vi "UI Main.vi"() -> ()   [LabVIEW 2018]
doc: "This is the main user interface for the LabVIEW Real-Time Sequencer."
uses:
  controls/UI Data.ctl
  controls/Configured Step.ctl
  controls/VI Reference Type.ctl
  controls/FPGA State.ctl
  Globals/Global - All UI Loop Stop.vi
  Globals/Global - UI Stream and Variable Connections.vi
  Globals/Global - Configuration Options.vi
  support/User Event - Stop/User Event - Stop.lvlib
  support/Message Queue/Message Queue.lvlib
panel:
  in  "Switch to Safe State":bool
  in  "Exit":bool
  out "System Status":string
  out "Current FPGA Control Mode":u16(ring) items=["Safe State", "Control (PID)"]
  in  "Settings Tab":T1(tab)
  in  "Build Sequence":bool
  in  "Control Sequence":i32(listbox)
  in  "Stop Sequence":bool
  in  "Pause":bool
  in  "Start":bool
  out "Output Values":cluster{dbl, dbl}(graph)
  out "Input Values":cluster{dbl, dbl}(graph)
  out "Actual Loop Period (ticks)":u32
  out "Largest Contiguous Memory (bytes)":dbl(graph)
  out "CPU Usage (%)":dbl(graph)
  out "Connected?":bool
  in  "Connect to Controller":bool
  in  "Controller Address":string
  # "LabVIEW Real-Time Sequencer"
  # "Connection Settings"
  # "Step Configuration Preview"
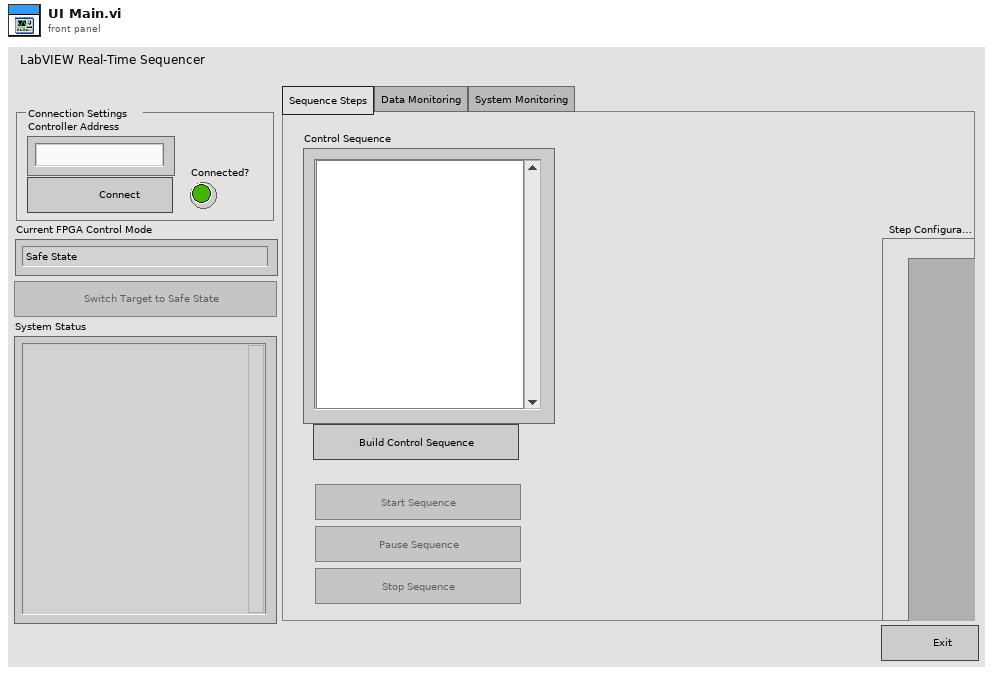
[diagram p1: front panel]
types:
  T1 = enum32{"Sequence Steps", "Data Monitoring", "System Monitoring"}
  T2 = typedef "VI Reference Type.ctl" = refnum<vi>
  T3 = typedef "Configured Step.ctl" = cluster{"Step Name":string, "Value":variant}
  T4 = typedef "UI Data.ctl" = cluster{"Switch to Safe State Ref":refnum<vi>, "Start Sequence Ref":refnum<vi>, "Pause Sequence Ref":refnum<vi>, "Stop Sequence Ref":refnum<vi>, "Build Sequence Ref":refnum<vi>, "SubPanel Ref":refnum<vi>}
  T5 = typedef "Message Queue.lvlib/All Message Queues.ctl" = cluster{"Sequencer Cmd Queue":refnum<queue>, "Vision Cmd Queue":refnum<queue>, "Motion Cmd Queue":refnum<queue>, "Message Handling Queue":refnum<queue>}
  T6 = typedef "FPGA State.ctl" = enum16{"Safe State", "Control (PID)"}
  T7 = typedef "Variable References.ctl" = cluster{"CPU Usage":refnum<k21>, "Contiguous Memory":refnum<k21>, "Input Values":refnum<k21>, "Output Values":refnum<k21>, "FPGA Mode":refnum<k21>, "Actual Loop Period":refnum<k21>}
  T8 = typedef "Raw Values.ctl" = cluster{"Channel 0":fxp<+/-,20,5>, "Channel 1":fxp<+/-,20,5>, "Channel 2":bool}
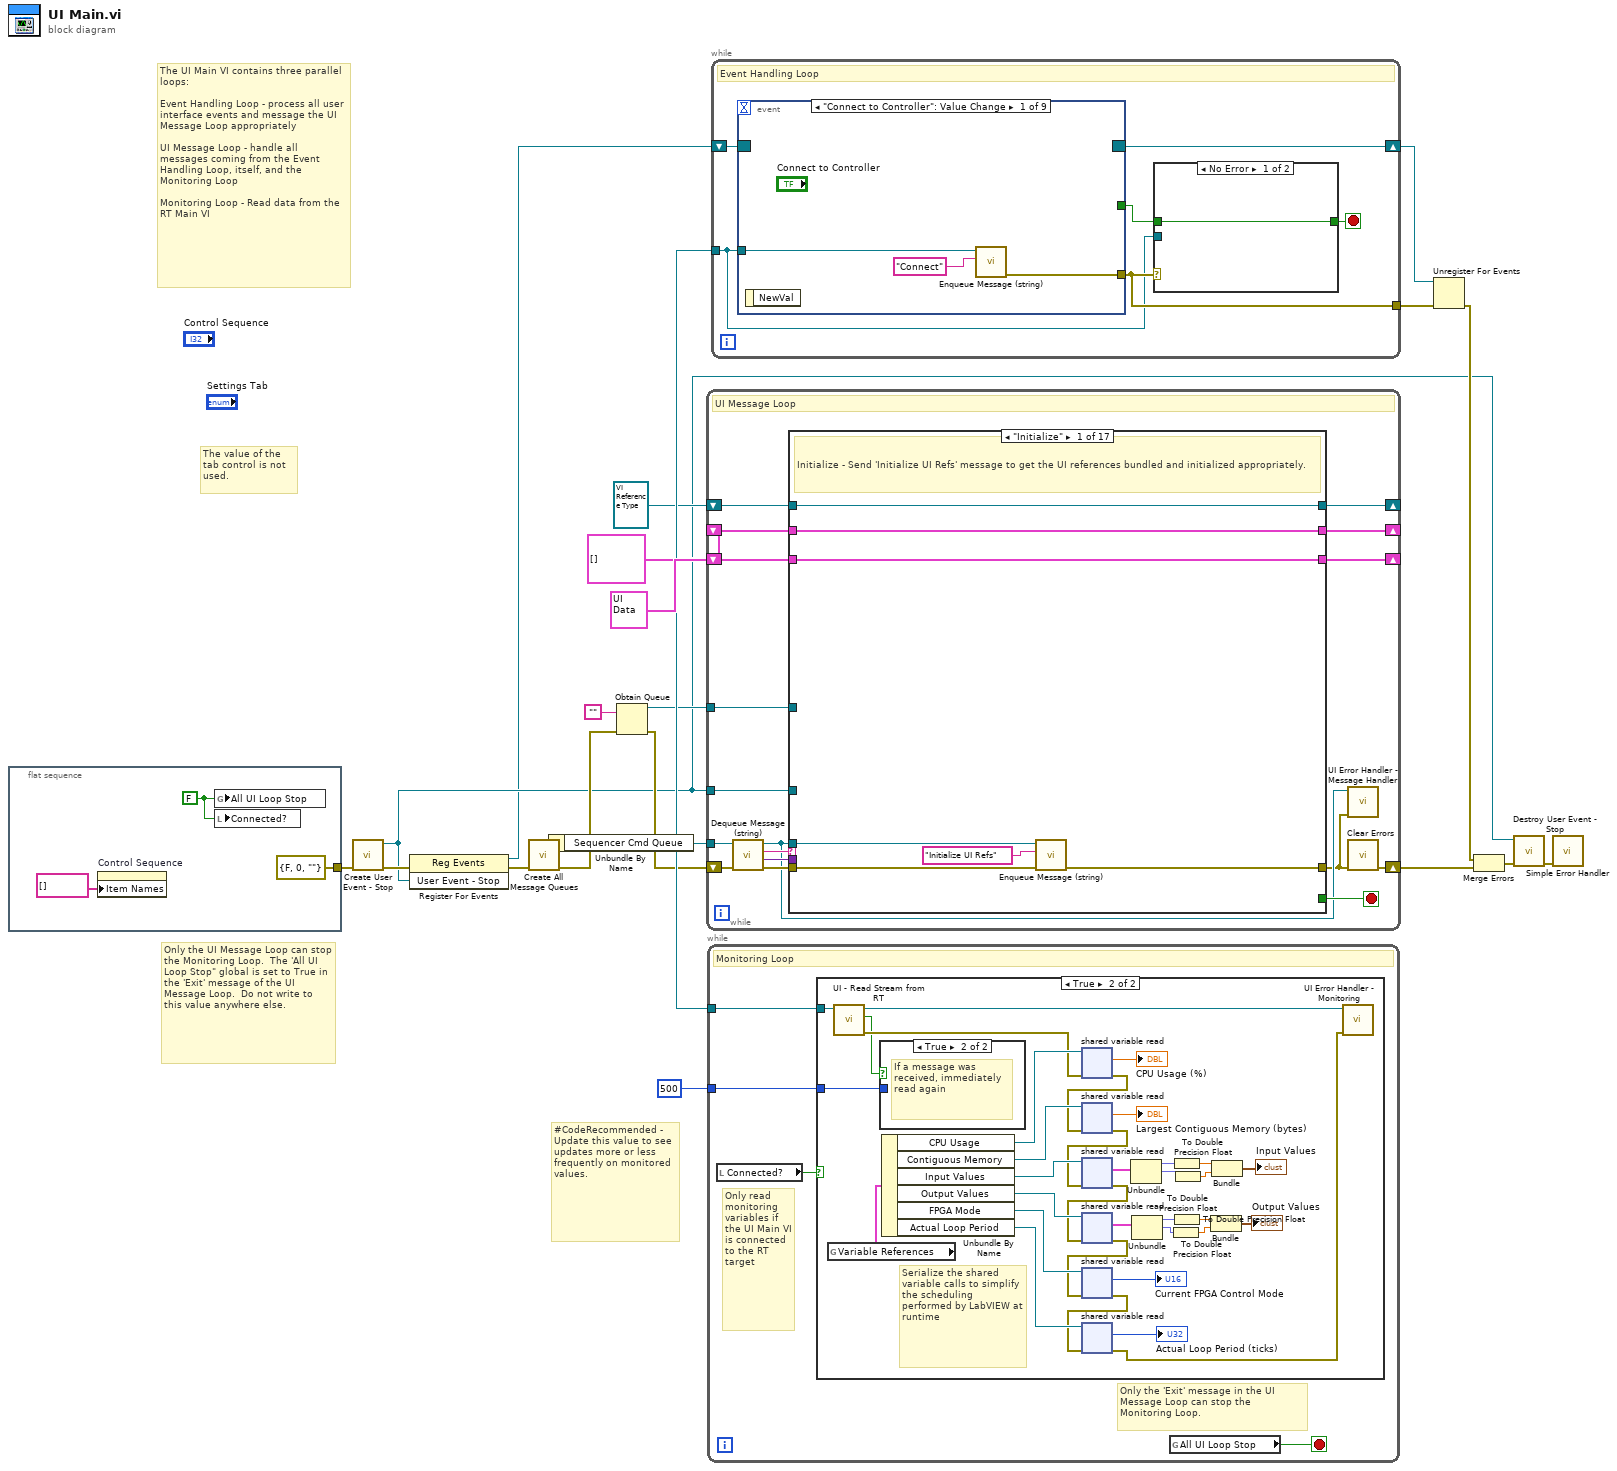
[diagram p0: block diagram]
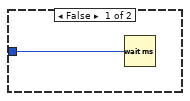
[diagram p2: hidden frame]
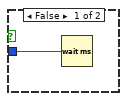
[diagram p3: hidden frame]
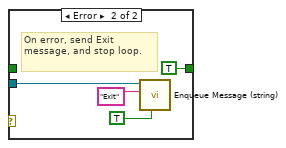
[diagram p4: hidden frame]
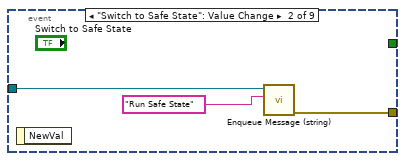
[diagram p5: hidden frame]
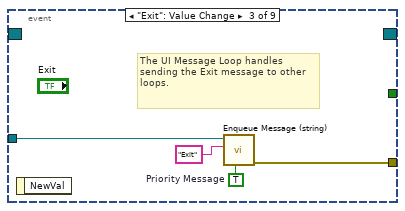
[diagram p6: hidden frame]
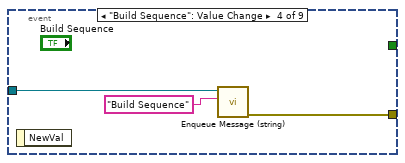
[diagram p7: hidden frame]
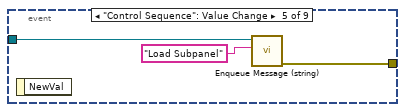
[diagram p8: hidden frame]
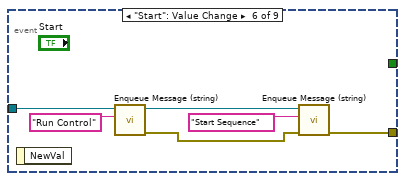
[diagram p9: hidden frame]
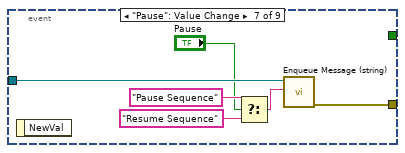
[diagram p10: hidden frame]
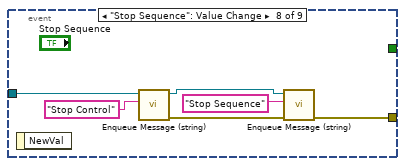
[diagram p11: hidden frame]
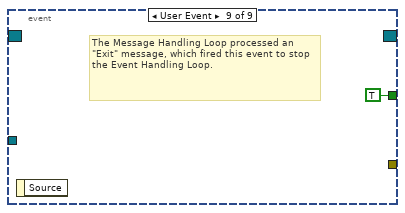
[diagram p12: hidden frame]
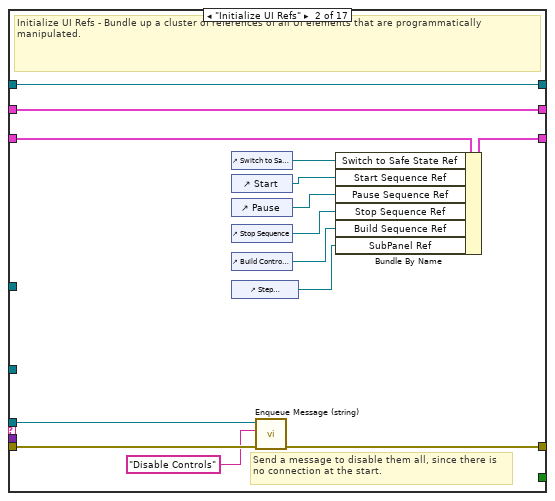
[diagram p13: hidden frame]
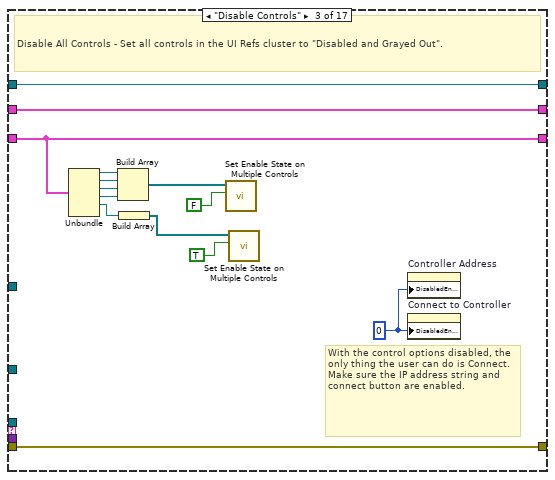
[diagram p14: hidden frame]
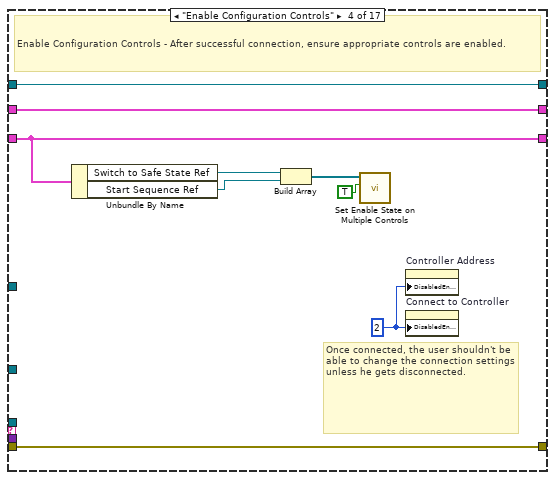
[diagram p15: hidden frame]
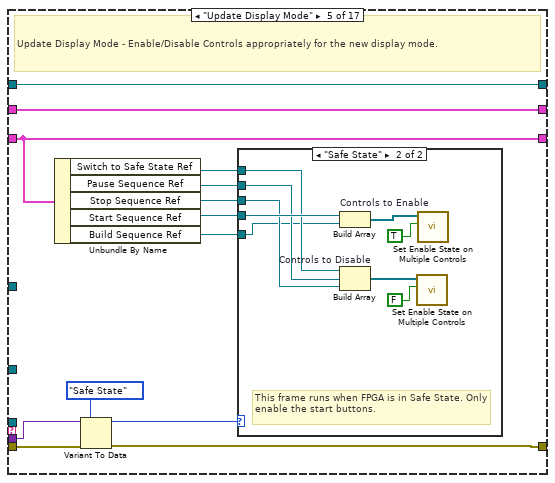
[diagram p16: hidden frame]
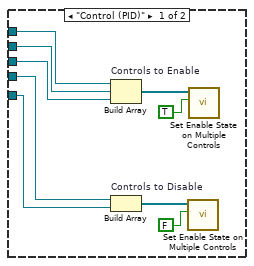
[diagram p17: hidden frame]
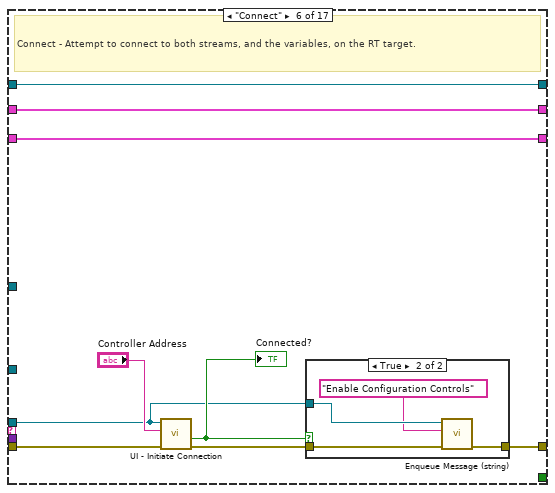
[diagram p18: hidden frame]
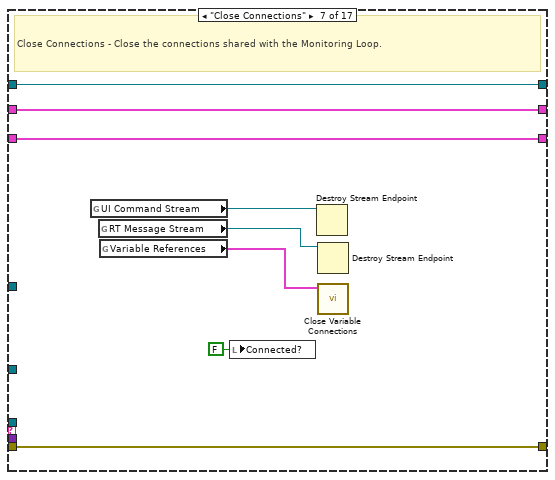
[diagram p20: hidden frame]
diagram:
  # "#CodeRecommended - Update this value to see updates more or less frequently on monitored values."
  # "The UI Main VI contains three parallel loops:\n\nEvent Handling Loop - process all user interface events and message the UI Message Loop appropriately\n\nUI Message Loop - handle all messages coming from the Event Handling Loop, itself, and the Monitoring Loop\n\nMonitoring Loop - Read data from the RT Main VI"
  # "The value of the tab control is not used."
  # "Only the UI Message Loop can stop the Monitoring Loop.  The 'All UI Loop Stop\" global is set to True in the 'Exit' message of the UI Message Loop.  Do not write to this value anywhere else."
  n1 = flat-sequence {
    tunnel: [errorcluster {"status"=FALSE, "code"=0, "source"=""} ("error in (no error)")] -> w12
    frame #0 {
      w23 = FALSE
      n2 = property on="Control Sequence" class="LstBox (strict)"("Item Names"=string[] []) -> ()  [unwired: 2 in, 2 out]
      n3 = global write "Global - All UI Loop Stop.vi" "All UI Loop Stop"(w23) -> ()
      n4 = local write "Connected?"(w23) -> ()
    }
  }
  n5 = call "Create User Event - Stop.vi"("error in (no error)"=w12) -> ("error out"=w4:errorcluster, "User Event - Stop"=w2:refnum<user-event>)  [unwired: 9 in]
  n6 = register-events(error in=w4, w2) -> (reference out=w1:refnum<event-registration>, error out=w3:errorcluster)  [unwired: 1 in]
  n7 = call "Create All Message Queues.vi"("error in (no error)"=w3) -> ("error out"=w6:errorcluster, "Message Queues out"=w18:T5)  [unwired: 9 in]
  n8 = Unbundle By Name(w18) -> ("Sequencer Cmd Queue"=w13:refnum<queue>)
  n9 = Obtain Queue(element data type="", error in (no error)=w6) -> (queue out=w7:refnum<queue>, error out=w5:errorcluster)  [unwired: 3 in, 1 out]
  n10 = while {
    tunnel: w13 -> [w35]
    tunnel: w2 -> [w40]
    shift-right: [w30] -> w21
    shift-left: w5 -> [w39]
    shift-right: [w33] -> _
    shift-left: T4 {"Switch to Safe State Ref"=refnum, "Start Sequence Ref"=refnum, "Pause Sequence Ref"=refnum, "Stop Sequence Ref"=refnum, "Build Sequence Ref"=refnum, "SubPanel Ref"=refnum} ("Measurement UI Controls") -> [w34]
    shift-right: [w29] -> _
    shift-left: T3[] [] ("Configured Steps Out") -> [w28]
    tunnel: w7 -> [w26]
    shift-right: [w25] -> _
    shift-left: T2 refnum ("VI reference") -> [w27]
    stop <- w41 stop-if-true
    # "UI Message Loop"
    n11 = call "Dequeue Message (string).vi"("error in (no error)"=w39, "Message Queue"=w35) -> ("error out"=w38:errorcluster, "Message Data"=w36:variant, "Message"=w37:string, "dup Message Queue"=w32:refnum<queue>)  [unwired: 6 in]
    n12 = case "Message Cases" shown="\"Initialize\"" w37 {
      selector: w37 -> [_ _ _ _ _ _ _ _ w150 _ _ w215 w260 _ _ _ w342]
      tunnel: w32 -> [w45 w58 _ _ _ w120 _ w142 w151 _ _ _ w264 _ w324 _ _]
      tunnel: w38 -> [w47 w62 w76 w80 w92 w125 w138 w144 w153 w172 w191 w219 w274 w300 w328 w335 _]
      tunnel: [w46 w59 w76 w80 w91 w119 w138 w143 w152 w171 w190 w218 w275 w298 w329 w334 w340] -> w31
      tunnel: [_ _ _ _ _ _ _ _ _ _ _ _ _ _ TRUE _ _] -> w41
      tunnel: w36 -> [_ _ _ _ w89 _ _ _ _ _ _ _ w272 w297 _ _ _]
      tunnel: w40 -> [_ _ _ _ _ _ _ _ _ _ _ _ _ _ w327 _ _]
      tunnel: w34 -> [w48 w56 w75 w82 w90 w124 w137 w146 w154 w174 w194 w221 w276 w299 w318 w333 w338]
      tunnel: [w48 w61 w75 w82 w90 w124 w137 w146 w154 w174 w194 w221 w276 w299 T4 {"Switch to Safe State Ref"=refnum, "Start Sequence Ref"=refnum, "Pause Sequence Ref"=refnum, "Stop Sequence Ref"=refnum, "Build Sequence Ref"=refnum, "SubPanel Ref"=refnum} ("Measurement UI Controls") w333 w338] -> w33
      tunnel: [w43 w50 w64 w78 w87 w118 w132 w140 w148 w176 w195 w216 w258 w289 w319 w332 w337] -> w29
      tunnel: w28 -> [w43 w50 w64 w78 w87 w118 w132 w140 w148 w175 w195 w216 w258 w289 w319 w332 w337]
      tunnel: w27 -> [w42 w49 w63 w77 w86 w117 w131 w139 w147 w169 w197 w217 w257 w288 w309 w331 w336]
      tunnel: w26 -> [_ _ _ _ _ _ _ _ _ w170 w198 _ _ _ w308 _ _]
      tunnel: [w42 w49 w63 w77 w86 w117 w131 w139 w147 T2 refnum ("VI Reference out") w196 w217 w257 w288 w309 w331 w336] -> w25
      frame "Initialize" {
        # "Initialize - Send 'Initialize UI Refs' message to get the UI references bundled and initialized appropriately."
        n13 = call "Enqueue Message (string).vi"("error in (no error)"=w47, "Message"="Initialize UI Refs", "Message Queue"=w45) -> ("error out"=w46:errorcluster)  [unwired: 7 in, 1 out]
      }
      frame "Initialize UI Refs" {
        # "Send a message to disable them all, since there is no connection at the start."
        # "Initialize UI Refs - Bundle up a cluster of references of all UI elements that are programmatically manipulated."
        n14 = control-ref of="Switch to Safe State"() -> (w60:refnum<vi>)
        n15 = control-ref of="Start"() -> (w55:refnum<vi>)
        n16 = control-ref of="Pause"() -> (w54:refnum<vi>)
        n17 = control-ref of="Stop Sequence"() -> (w53:refnum<vi>)
        n18 = control-ref of="Build Control Sequence"() -> (w52:refnum<vi>)
        n19 = control-ref of="Step Configuration Information"() -> (w51:refnum<vi>)
        n20 = call "Enqueue Message (string).vi"("error in (no error)"=w62, "Message"="Disable Controls", "Message Queue"=w58) -> ("error out"=w59:errorcluster)  [unwired: 7 in, 1 out]
        n21 = Bundle By Name(cluster=w56, "Switch to Safe State Ref"=w60, "Start Sequence Ref"=w55, "Pause Sequence Ref"=w54, "Stop Sequence Ref"=w53, "Build Sequence Ref"=w52, "SubPanel Ref"=w51) -> (w61:T4)
      }
      frame "Disable Controls" {
        w68 = 0
        # "With the control options disabled, the only thing the user can do is Connect. Make sure the IP address string and connect button are enabled."
        # "Disable All Controls - Set all controls in the UI Refs cluster to \"Disabled and Grayed Out\"."
        n22 = Unbundle(w75) -> ("Switch to Safe State Ref"=w74:refnum<vi>, "Start Sequence Ref"=w73:refnum<vi>, "Pause Sequence Ref"=w72:refnum<vi>, "Stop Sequence Ref"=w71:refnum<vi>, "Build Sequence Ref"=w66:refnum<vi>)  [unwired: 1 out]
        n23 = Build Array(w74, w73, w72, w71) -> (w70:refnum<vi>[])
        n24 = Build Array(w66) -> (w65:refnum<vi>[])
        n25 = call "Set Enable State on Multiple Controls.vi"("Enable?"=FALSE, "Controls"=w70) -> ()  [unwired: 10 in]
        n26 = call "Set Enable State on Multiple Controls.vi"("Enable?"=TRUE, "Controls"=w65) -> ()  [unwired: 10 in]
        n27 = property on="Controller Address" class="Str"("DisabledEnum"=w68) -> ()  [unwired: 2 in, 2 out]
        n28 = property on="Connect to Controller" class="Bool"("DisabledEnum"=w68) -> ()  [unwired: 2 in, 2 out]
      }
      frame "Enable Configuration Controls" {
        w83 = 2
        # "Once connected, the user shouldn't be able to change the connection settings unless he gets disconnected."
        # "Enable Configuration Controls - After successful connection, ensure appropriate controls are enabled."
        n29 = Unbundle By Name(w82) -> ("Switch to Safe State Ref"=w81:refnum<vi>, "Start Sequence Ref"=w79:refnum<vi>)
        n30 = Build Array(w81, w79) -> (w85:refnum<vi>[])
        n31 = call "Set Enable State on Multiple Controls.vi"("Enable?"=TRUE, "Controls"=w85) -> ()  [unwired: 10 in]
        n32 = property on="Controller Address" class="Str"("DisabledEnum"=w83) -> ()  [unwired: 2 in, 2 out]
        n33 = property on="Connect to Controller" class="Bool"("DisabledEnum"=w83) -> ()  [unwired: 2 in, 2 out]
      }
      frame "Update Display Mode" {
        # "Update Display Mode - Enable/Disable Controls appropriately for the new display mode."
        n34 = Unbundle By Name(w90) -> ("Switch to Safe State Ref"=w97:refnum<vi>, "Pause Sequence Ref"=w96:refnum<vi>, "Stop Sequence Ref"=w95:refnum<vi>, "Start Sequence Ref"=w94:refnum<vi>, "Build Sequence Ref"=w88:refnum<vi>)
        n35 = Variant To Data(error in=w92, type=FPGA_State."Safe State" ("FPGA State"), Variant=w89) -> (data=w98:T6, error out=w91:errorcluster)
        n36 = case shown="\"Safe State\"" w98 {
          tunnel: w97 -> [w103 w111]
          tunnel: w96 -> [w101 w109]
          tunnel: w95 -> [w100 w110]
          tunnel: w94 -> [w102 w112]
          tunnel: w88 -> [w99 w108]
          frame "Control (PID)" {
            n37 = Build Array "Controls to Enable"(w103, w101, w100) -> (w107:refnum<vi>[])
            n38 = Build Array "Controls to Disable"(w102, w99) -> (w105:refnum<vi>[])
            n39 = call "Set Enable State on Multiple Controls.vi"("Enable?"=FALSE, "Controls"=w105) -> ()  [unwired: 10 in]
            n40 = call "Set Enable State on Multiple Controls.vi"("Enable?"=TRUE, "Controls"=w107) -> ()  [unwired: 10 in]
          }
          frame "Safe State" {
            # "This frame runs when FPGA is in Safe State. Only enable the start buttons."
            n41 = Build Array "Controls to Enable"(w112, w108) -> (w116:refnum<vi>[])
            n42 = Build Array "Controls to Disable"(w111, w109, w110) -> (w114:refnum<vi>[])
            n43 = call "Set Enable State on Multiple Controls.vi"("Enable?"=FALSE, "Controls"=w114) -> ()  [unwired: 10 in]
            n44 = call "Set Enable State on Multiple Controls.vi"("Enable?"=TRUE, "Controls"=w116) -> ()  [unwired: 10 in]
          }
        }
      }
      frame "Connect" {
        # "Connect - Attempt to connect to both streams, and the variables, on the RT target."
        n45 = call "UI - Initiate Connection.vi"("error in (no error)"=w125, "Controller Address"="Controller Address", "Message Queue"=w120) -> ("error out"=w122:errorcluster, "Connected?"=w121:bool)  [unwired: 7 in]
        "Connected?" <- w121
        n46 = case shown="True" w121 {
          tunnel: w122 -> [w126 w130]
          tunnel: w120 -> [_ w129]
          tunnel: [w126 w128] -> w119
          frame False {
          }
          frame True {
            n47 = call "Enqueue Message (string).vi"("error in (no error)"=w130, "Message"="Enable Configuration Controls", "Message Queue"=w129) -> ("error out"=w128:errorcluster)  [unwired: 7 in, 1 out]
          }
        }
      }
      frame "Close Connections" {
        # "Close Connections - Close the connections shared with the Monitoring Loop."
        n48 = global read "Global - UI Stream and Variable Connections.vi" "UI Command Stream"() -> (w136:refnum<k21>)
        n49 = global read "Global - UI Stream and Variable Connections.vi" "RT Message Stream"() -> (w135:refnum<k21>)
        n50 = global read "Global - UI Stream and Variable Connections.vi" "Variable References"() -> (w134:T7)
        n51 = local write "Connected?"(FALSE ("Connected?")) -> ()
        n52 = Destroy Stream Endpoint(11:w136) -> ()  [unwired: 1 in, 1 out]
        n53 = Destroy Stream Endpoint(11:w135) -> ()  [unwired: 1 in, 1 out]
        n54 = call "Close Variable Connections.vi"("Variable References"=w134) -> ()  [unwired: 11 in]
      }
      frame "Disconnect UI" {
        # "Disconnect UI - Something has gone wrong with the connection. Reinitialize the UI to its disconnected state."
        n55 = local write "Connected?"(FALSE ("Connected?")) -> ()
        n56 = call "Enqueue Message (string).vi"("error in (no error)"=w144, "Message"="Disable Controls", "Message Queue"=w142) -> ("error out"=w143:errorcluster)  [unwired: 7 in, 1 out]
      }
      frame "Run Control", "Run Safe State", "Stop Control" {
        # "Run/Stop buttons - Send a command to switch the FPGA into the appropriate state. Send a message to update this UI to reflect the new state."
        n57 = local read "Connected?"() -> (w149:bool)
        n58 = case shown="True" w149 {
          tunnel: w153 -> [w155 w165]
          tunnel: [w155 w161] -> w152
          tunnel: w151 -> [_ w160]
          tunnel: w150 -> [_ w159]
          frame False {
            # "Don't bother trying to send a message to the RT system if UI Main VI isn't even connected"
          }
          frame True {
            # "Run Control switch into PID control state. Anything else switches to Safe State."
            n59 = case shown="\"Safe State\", \"Stop Control\", Default" w159 {
              tunnel: [FPGA_State."Safe State" ("FPGA State") FPGA_State."Control (PID)" ("FPGA State")] -> w156
              frame "Safe State", "Stop Control", Default {
              }
              frame "Run Control" {
              }
            }
            n60 = global read "Global - UI Stream and Variable Connections.vi" "UI Command Stream"() -> (w157:refnum<k21>)
            n61 = Bundle("Update FPGA State", "FPGA State"=w156) -> (w162:cluster{string, "FPGA State":T6})  [unwired: 1 in]
            n62 = shared-variable-write(w157, w165, w162) -> (w164:errorcluster)  [unwired: 1 in, 2 out]
            n63 = call "Enqueue Message (string).vi"("error in (no error)"=w164, "Message Data"=w156, "Message"="Update Display Mode", "Message Queue"=w160) -> ("error out"=w161:errorcluster)  [unwired: 6 in, 1 out]
          }
        }
      }
      frame "Build Sequence" {
        # "The subpanel must be unloaded because the VIs used in the subpanel are also used the 'Build Control Sequence' dialog and cannot be loaded in two subpanels simultaneously."
        # "Retrieve the step names to display them in the 'Control Sequence' listbox."
        # "Build Sequence - Stop and unload the VI running in the subpanel, if one exists. Then open the 'Build Control Sequence' dialog that allows the user to build, configure, and modify the control sequence."
        n64 = Not A Number/Path/Refnum?(number/path/refnum=w169) -> (NaN/Path/Refnum?=w177:bool)
        n65 = Unbundle By Name(w174) -> ("SubPanel Ref"=w173:refnum<vi>)
        n66 = case shown="False" w177 {
          tunnel: [w186 w187] -> w178
          tunnel: w172 -> [w185 w187]
          tunnel: w170 -> [w184 _]
          tunnel: w169 -> [w183 _]
          frame False {
            n67 = call "Stop Configuration VI.vi"("error in (no error)"=w185, "Subpanel Queue In"=w184, "VI in"=w183) -> ("error out"=w186:errorcluster)  [unwired: 6 in, 2 out]
          }
          frame True {
          }
        }
        n68 = invoke class="SubPnl" method="Remove VI"(reference=w173, error in=w178) -> (error out=w179:errorcluster)  [unwired: 1 in, 2 out]
        n69 = call "Build Test Sequence.vi"("error in"=w179, "Configured Steps In"=w175) -> ("error out"=w180:errorcluster, "Configured Steps Out"=w176:T3[])  [unwired: 8 in]
        n70 = for {
          tunnel: w176 -> [w189] mode=indexing
          tunnel: [w188] -> w182 mode=indexing
          n71 = Unbundle(w189) -> ("Step Name"=w188:string)  [unwired: 1 out]
        }
        n72 = property on="Control Sequence" class="LstBox (strict)"(error in=w180, "Item Names"=w182, "Val(Sgnl)"=0 ("Value (Signaling)")) -> (error out=w171:errorcluster)  [unwired: 1 in, 1 out]
      }
      frame "Load Subpanel" {
        # "Load Subpanel - Stop and unload the VI currently running in the subpanel and load/initialize the VI associated with the currently selected control step."
        n73 = Not A Number/Path/Refnum?(number/path/refnum=w197) -> (NaN/Path/Refnum?=w206:bool)
        n74 = case shown="False" w206 {
          tunnel: w197 -> [w212 _]
          tunnel: [w211 w213] -> w200
          tunnel: w198 -> [w210 w214]
          tunnel: [w209 w214] -> w201
          tunnel: w191 -> [w208 w213]
          frame False {
            n75 = call "Stop Configuration VI.vi"("error in (no error)"=w208, "Subpanel Queue In"=w210, "VI in"=w212) -> ("error out"=w211:errorcluster, "Subpanel Queue Out"=w209:refnum<queue>)  [unwired: 6 in, 1 out]
          }
          frame True {
          }
        }
        n76 = Unbundle By Name(w194) -> ("SubPanel Ref"=w193:refnum<vi>)
        n77 = property on="Control Sequence" class="LstBox (strict)"(error in=w200) -> (error out=w199:errorcluster, "Item Names"=w207:string[], "Value"=w202:i32)  [unwired: 1 in, 1 out]
        n78 = invoke class="SubPnl" method="Remove VI"(reference=w193, error in=w199) -> (reference out=w192:refnum<vi>, error out=w205:errorcluster)  [unwired: 1 in, 1 out]
        n79 = Index Array(array=w207, index=w202) -> (element=w203:string)
        n80 = call "Initialize Configuration VI.vi"("Step Number"=w202, "Step Name"=w203, "error in (no error)"=w205, "Subpanel Queue in"=w201, "Configured Steps In"=w195) -> ("error out"=w204:errorcluster, "VI Reference out"=w196:T2)  [unwired: 4 in, 1 out]
        n81 = invoke on="Invoke Node" class="SubPnl" method="Insert VI"(reference=w192, error in=w204, "VI Ref"=w196) -> (error out=w190:errorcluster)  [unwired: 1 in, 3 out]
      }
      frame "Pause Sequence", "Resume Sequence", "Start Sequence", "Stop Sequence" {
        # "Start/Stop/Pause/Resume Sequence - Send a command to the RT target to start/stop/pause/resume the control sequence."
        n82 = local read "Connected?"() -> (w220:bool)
        n83 = case shown="True" w220 {
          tunnel: w219 -> [w222 w225]
          tunnel: [w222 w224] -> w218
          tunnel: w216 -> [_ w223]
          tunnel: w215 -> [_ w226]
          frame False {
            # "Do not send a message to the RT system if UI Main VI is not connected."
          }
          frame True {
            # "Send the configured control steps with the \"Start Sequence\" command; otherwise, the message data is empty."
            n84 = case shown="\"Start Sequence\"" w226 {
              selector: w226 -> [_ _ _ _ w253]
              tunnel: w225 -> [w229 w236 w241 w246 _]
              tunnel: [w228 w235 w240 w245 w252] -> w224
              tunnel: w223 -> [_ _ _ w247 _]
              frame "Pause Sequence" {
                n85 = global read "Global - UI Stream and Variable Connections.vi" "UI Command Stream"() -> (w232:refnum<k21>)
                n86 = Bundle("Pause Sequence", "variant"=variant) -> (w231:cluster{string, "variant":variant})  [unwired: 1 in]
                n87 = shared-variable-write(w232, w229, w231) -> (w228:errorcluster)  [unwired: 1 in, 2 out]
              }
              frame "Resume Sequence" {
                n88 = global read "Global - UI Stream and Variable Connections.vi" "UI Command Stream"() -> (w234:refnum<k21>)
                n89 = Bundle("Resume Sequence", "variant"=variant) -> (w238:cluster{string, "variant":variant})  [unwired: 1 in]
                n90 = shared-variable-write(w234, w236, w238) -> (w235:errorcluster)  [unwired: 1 in, 2 out]
              }
              frame "Stop Sequence" {
                n91 = global read "Global - UI Stream and Variable Connections.vi" "UI Command Stream"() -> (w243:refnum<k21>)
                n92 = Bundle("Stop Sequence", "variant"=variant) -> (w244:cluster{string, "variant":variant})  [unwired: 1 in]
                n93 = shared-variable-write(w243, w241, w244) -> (w240:errorcluster)  [unwired: 1 in, 2 out]
              }
              frame "Start Sequence" {
                n94 = global read "Global - UI Stream and Variable Connections.vi" "UI Command Stream"() -> (w251:refnum<k21>)
                n95 = To Variant(anything=w247) -> (Variant=w249:variant)
                n96 = Bundle("Start Sequence", "Variant"=w249) -> (w250:cluster{string, "Variant":variant})  [unwired: 1 in]
                n97 = shared-variable-write(w251, w246, w250) -> (w245:errorcluster)  [unwired: 1 in, 2 out]
              }
              frame Default {
                n98 = Format Into String(format string="The invalid message string \"%s\" was received in the Message Handling Loop." ("Invalid Message Loop Message"), w253) -> (resulting string=w254:string)  [unwired: 2 in, 1 out]
                n99 = call <vilib>:"Error Cluster From Error Code.vi"("error message (\"\")"=w254, "error code (0)"=1) -> ("error out"=w252:errorcluster)  [unwired: 7 in]
              }
            }
          }
        }
      }
      frame "Critical Error", "Log-Only Error", "Non-Critical Error", "RT Error" {
        # "Error - Display message in status indicator on panel.  If it's a critical error, shut down this VI with an 'Exit' message."
        n100 = case shown="Default" w260 {
          selector: w260 -> [_ w278]
          tunnel: ["UI Error" w278] -> w259
          frame Default {
          }
          frame "RT Error" {
          }
        }
        n101 = Variant To Data(error in=w274, type=errorcluster {"status"=FALSE, "code"=0, "source"=""} ("error constant"), Variant=w272) -> (data=w267:errorcluster, error out=w273:errorcluster)
        n102 = Unbundle By Name(w267) -> ("code"=w266:i32, "source"=w270:string)
        n103 = Format Date/Time String() -> (date/time string=w269:string)  [unwired: 3 in]
        n104 = Format Into String(format string="\n%s: %s %d - %s", w269, w259, w266, w270) -> (resulting string=w261:string)  [unwired: 2 in, 1 out]
        n105 = call "Enqueue Message (string).vi"("error in (no error)"=w273, "Message Data"=w261, "Message"="Update System Status", "Message Queue"=w264) -> ("error out"=w265:errorcluster, "dup Message Queue"=w263:refnum<queue>)  [unwired: 6 in]
        n106 = case shown="\"Critical Error\"" w260 {
          tunnel: w265 -> [w279 w283]
          tunnel: w263 -> [_ w281]
          tunnel: [w279 w282] -> w275
          frame Default {
          }
          frame "Critical Error" {
            n107 = call "Enqueue Message (string).vi"("error in (no error)"=w283, "Message"="Exit", "Message Queue"=w281) -> ("error out"=w282:errorcluster)  [unwired: 7 in, 1 out]
          }
        }
      }
      frame "Update System Status" {
        # "#CodeRecommended - The code below ensures that the System Status string value does not become too large.  It uses the same maximum size as the RT error log to determine whether or not to remove the last half of the log string. Change this logic if you wish to maintain more/less of the information in the System Status string."
        # "Update System Status - Add a new string to the beginning of the System Status string on the UI."
        n108 = Variant To Data(error in=w300, type="", Variant=w297) -> (data=w284:string, error out=w298:errorcluster)
        n109 = local read "System Status"() -> (w293:string)
        n110 = global read "Global - Configuration Options.vi" "Error Log Max Size (bytes)"() -> (w291:i64)
        n111 = String Length(string=w293) -> (length=w294:i32)
        n112 = Concatenate Strings("===" ("string"), w284, "\r") -> (w285:string)
        n113 = Greater?(x=w294, y=w291) -> (0:w292:bool)
        n114 = case shown="False" w292 {
          tunnel: w293 -> [w301 w305]
          tunnel: w291 -> [_ w304]
          tunnel: [w301 w306] -> w290
          frame False {
          }
          frame True {
            n115 = Divide(x=w304, y=i64 2) -> (x/y=w303:dbl)
            n116 = String Subset(string=w305, length (rest)=w303) -> (substring=w306:string)  [unwired: 1 in]
          }
        }
        n117 = Concatenate Strings(w285, w290) -> (→"System Status":string)
      }
      frame "Exit" {
        # "Release the subpanel queue reference"
        # "Close all connections"
        # "Stop Monitoring Loop"
        # "Stop Event Handling Loop"
        # "Release the UI Message queue reference"
        # "Stop UI Message Loop"
        # "Exit - Fire the User Event to stop the Event Handling Loop, and toggle the local variable to stop the Monitoring Loop.  This message alone causes all three loops to stop."
        n118 = Release Queue(queue=w308) -> (error out=w307:errorcluster)  [unwired: 2 in, 2 out]
        n119 = global write "Global - All UI Loop Stop.vi" "All UI Loop Stop"(TRUE ("Stop Monitoring Loop")) -> ()
        n120 = call "Fire User Event - Stop.vi"("User Event - Stop"=w327) -> ("error out"=w326:errorcluster)  [unwired: 10 in]
        n121 = Unbundle(w318) -> ("Switch to Safe State Ref"=w317:refnum<vi>, "Start Sequence Ref"=w316:refnum<vi>, "Pause Sequence Ref"=w315:refnum<vi>, "Stop Sequence Ref"=w314:refnum<vi>, "Build Sequence Ref"=w313:refnum<vi>, "SubPanel Ref"=w312:refnum<vi>)
        n122 = Release Queue(queue=w324, error in (no error)=w328) -> (error out=w325:errorcluster)  [unwired: 1 in, 2 out]
        n123 = Build Array(w317, w316, w315, w314, w313, w312) -> (w311:refnum<vi>[])
        n124 = Close Reference(reference=w311) -> ()  [unwired: 1 in, 1 out]
        n125 = global read "Global - UI Stream and Variable Connections.vi" "UI Command Stream"() -> (w322:refnum<k21>)
        n126 = global read "Global - UI Stream and Variable Connections.vi" "RT Message Stream"() -> (w321:refnum<k21>)
        n127 = global read "Global - UI Stream and Variable Connections.vi" "Variable References"() -> (w320:T7)
        n128 = Destroy Stream Endpoint(11:w322) -> ()  [unwired: 1 in, 1 out]
        n129 = Destroy Stream Endpoint(11:w321) -> ()  [unwired: 1 in, 1 out]
        n130 = call "Close Variable Connections.vi"("Variable References"=w320) -> ()  [unwired: 11 in]
        n131 = Merge Errors(w307, w326, w325) -> (w329:errorcluster)
      }
      frame "---Copy This Frame---" {
        # "Duplicate this frame when creating new messages.  Change this comment in the duplicated frame to describe this message."
        n132 = Merge Errors(w335) -> (w334:errorcluster)
      }
      frame Default {
        # "'Default' case only runs if there is a message that isn't defined in any of the other cases.  Output a programming error."
        n133 = Format Into String(format string="The invalid message string \"%s\" was received in the Message Handling Loop." ("Invalid Message Loop Message"), w342) -> (resulting string=w339:string)  [unwired: 2 in, 1 out]
        n134 = call <vilib>:"Error Cluster From Error Code.vi"("error message (\"\")"=w339, "error code (0)"=1) -> ("error out"=w340:errorcluster)  [unwired: 7 in]
      }
    }
    n135 = call "UI Error Handler - Message Handler.vi"("error in (no error)"=w31, "Message Queue"=w32) -> ()  [unwired: 9 in, 1 out]
    n136 = call <vilib>:"Clear Errors.vi"("error in (no error)"=w31) -> ("error out"=w30:errorcluster)  [unwired: 5 in, 1 out]
  }
  n137 = while {
    tunnel: w13 -> [w346]
    tunnel: u32 500 ("milliseconds to wait") -> [w344]
    stop <- w347 stop-if-true
    # "Only read monitoring variables if the UI Main VI is connected to the RT target"
    # "Only the 'Exit' message in the UI Message Loop can stop the Monitoring Loop."
    # "Monitoring Loop"
    n138 = local read "Connected?"() -> (w345:bool)
    n139 = case shown="True" w345 {
      tunnel: w346 -> [_ w366]
      tunnel: w344 -> [w348 w361]
      frame False {
        n140 = Wait (ms)(milliseconds to wait=w348) -> ()  [unwired: 1 out]
      }
      frame True {
        # "Serialize the shared variable calls to simplify the scheduling performed by LabVIEW at runtime"
        n141 = global read "Global - UI Stream and Variable Connections.vi" "Variable References"() -> (w364:T7)
        n142 = call "UI - Read Stream from RT.vi"("Message Queue"=w366) -> ("error out"=w372:errorcluster, "Message Received?"=w362:bool, "dup Message Queue"=w365:refnum<queue>)  [unwired: 8 in]
        n143 = case shown="True" w362 {
          tunnel: w361 -> [w383 _]
          frame False {
            n144 = Wait (ms)(milliseconds to wait=w383) -> ()  [unwired: 1 out]
          }
          frame True {
            # "If a message was received, immediately read again"
          }
        }
        n145 = Unbundle By Name(w364) -> ("CPU Usage"=w379:refnum<k21>, "Contiguous Memory"=w378:refnum<k21>, "Input Values"=w377:refnum<k21>, "Output Values"=w376:refnum<k21>, "FPGA Mode"=w375:refnum<k21>, "Actual Loop Period"=w374:refnum<k21>)
        n146 = shared-variable-read(w379, w372) -> (w371:errorcluster, →"CPU Usage (%)":dbl)  [unwired: 2 out]
        n147 = shared-variable-read(w378, w371) -> (w370:errorcluster, →"Largest Contiguous Memory (bytes)":dbl)  [unwired: 2 out]
        n148 = shared-variable-read(w377, w370) -> (w369:errorcluster, w360:T8)  [unwired: 2 out]
        n149 = shared-variable-read(w376, w369) -> (w368:errorcluster, w355:T8)  [unwired: 2 out]
        n150 = shared-variable-read(w375, w368) -> (w367:errorcluster, →"Current FPGA Control Mode":T6)  [unwired: 2 out]
        n151 = shared-variable-read(w374, w367) -> (w373:errorcluster, →"Actual Loop Period (ticks)":u32)  [unwired: 2 out]
        n152 = Unbundle(w360) -> ("Channel 0"=w359:fxp<+/-,20,5>, "Channel 1"=w358:fxp<+/-,20,5>)  [unwired: 1 out]
        n153 = Unbundle(w355) -> ("Channel 0"=w354:fxp<+/-,20,5>, "Channel 1"=w353:fxp<+/-,20,5>)  [unwired: 1 out]
        n154 = To Double Precision Float(number=w353) -> (double precision float=w351:dbl)
        n155 = To Double Precision Float(number=w359) -> (double precision float=w357:dbl)
        n156 = To Double Precision Float(number=w354) -> (double precision float=w352:dbl)
        n157 = To Double Precision Float(number=w358) -> (double precision float=w356:dbl)
        n158 = Bundle(w352, w351) -> (→"Output Values":cluster{dbl, dbl})  [unwired: 1 in]
        n159 = Bundle(w357, w356) -> (→"Input Values":cluster{dbl, dbl})  [unwired: 1 in]
        n160 = call "UI Error Handler - Monitoring.vi"("error in (no error)"=w373, "Message Queue"=w365) -> ()  [unwired: 9 in, 1 out]
      }
    }
    n161 = global read "Global - All UI Loop Stop.vi" "All UI Loop Stop"() -> (w347:bool)
  }
  n162 = while {
    tunnel: w13 -> [w385]
    tunnel: [w387] -> w20
    shift-right: [w384] -> w16
    shift-left: w1 -> [w386]
    stop <- w388 stop-if-true
    # "Event Handling Loop"
    n163 = event shown="[0] \"Connect to Controller\": Value Change" {
      selector: w386 -> [_ _ _ _ _ _ _ _ _]
      dyn-events: [_ _ _ _ _ _ _ _ _] -> w384
      timeout: _ -> [_ _ _ _ _ _ _ _ _]
      tunnel: [_ _ _ _ _ _ _ _ TRUE ("Discard?")] -> w389
      tunnel: w385 -> [w395 w398 w401 w407 w409 w413 w422 w425 _]
      tunnel: [w397 w400 w404 w405 w408 w415 w421 w427 _] -> w387
      event "Connect to Controller": Value Change {
        n164 = event-data() -> ()  [unwired: 1 in, 1 out]
        n165 = call "Enqueue Message (string).vi"("Message"="Connect", "Message Queue"=w395) -> ("error out"=w397:errorcluster)  [unwired: 8 in, 1 out]
      }
      event "Switch to Safe State": Value Change {
        n166 = event-data() -> ()  [unwired: 1 in, 1 out]
        n167 = call "Enqueue Message (string).vi"("Message"="Run Safe State", "Message Queue"=w398) -> ("error out"=w400:errorcluster)  [unwired: 8 in, 1 out]
      }
      event "Exit": Value Change {
        w402 = TRUE  # Priority Message
        # "The UI Message Loop handles sending the Exit message to other loops."
        n168 = event-data() -> ()  [unwired: 1 in, 1 out]
        n169 = call "Enqueue Message (string).vi"("Priority Message? (F)"=w402, "Message"="Exit", "Message Queue"=w401) -> ("error out"=w404:errorcluster)  [unwired: 7 in, 1 out]
      }
      event "Build Sequence": Value Change {
        n170 = event-data() -> ()  [unwired: 1 in, 1 out]
        n171 = call "Enqueue Message (string).vi"("Message"="Build Sequence", "Message Queue"=w407) -> ("error out"=w405:errorcluster)  [unwired: 8 in, 1 out]
      }
      event "Control Sequence": Value Change {
        n172 = event-data() -> ()  [unwired: 1 in, 1 out]
        n173 = call "Enqueue Message (string).vi"("Message"="Load Subpanel", "Message Queue"=w409) -> ("error out"=w408:errorcluster)  [unwired: 8 in, 1 out]
      }
      event "Start": Value Change {
        n174 = event-data() -> ()  [unwired: 1 in, 1 out]
        n175 = call "Enqueue Message (string).vi"("Message"="Run Control", "Message Queue"=w413) -> ("error out"=w411:errorcluster, "dup Message Queue"=w412:refnum<queue>)  [unwired: 8 in]
        n176 = call "Enqueue Message (string).vi"("error in (no error)"=w411, "Message"="Start Sequence", "Message Queue"=w412) -> ("error out"=w415:errorcluster)  [unwired: 7 in, 1 out]
      }
      event "Pause": Value Change {
        n177 = event-data() -> ()  [unwired: 1 in, 1 out]
        n178 = Select(t="Pause Sequence" ("Message"), s="Pause", f="Resume Sequence") -> (s? t:f=w419:string)
        n179 = call "Enqueue Message (string).vi"("Message"=w419, "Message Queue"=w422) -> ("error out"=w421:errorcluster)  [unwired: 8 in, 1 out]
      }
      event "Stop Sequence": Value Change {
        n180 = event-data() -> ()  [unwired: 1 in, 1 out]
        n181 = call "Enqueue Message (string).vi"("Message"="Stop Control", "Message Queue"=w425) -> ("error out"=w423:errorcluster, "dup Message Queue"=w424:refnum<queue>)  [unwired: 8 in]
        n182 = call "Enqueue Message (string).vi"("error in (no error)"=w423, "Message"="Stop Sequence", "Message Queue"=w424) -> ("error out"=w427:errorcluster)  [unwired: 7 in, 1 out]
      }
      event User Event {
        # "The Message Handling Loop processed an \"Exit\" message, which fired this event to stop the Event Handling Loop."
        n183 = event-data() -> ()  [unwired: 1 in, 1 out]
      }
    }
    n184 = case shown="No Error" w387 {
      tunnel: [w390 TRUE ("Discard?")] -> w388
      tunnel: w389 -> [w390 _]
      tunnel: w385 -> [_ w391]
      frame No Error {
      }
      frame Error {
        # "On error, send Exit message, and stop loop."
        n185 = call "Enqueue Message (string).vi"("Priority Message? (F)"=TRUE ("Discard?"), "Message"="Exit", "Message Queue"=w391) -> ()  [unwired: 7 in, 2 out]
      }
    }
  }
  n186 = Unregister For Events(event registration refnum=w16, error in=w20) -> (error out=w17:errorcluster)
  n187 = Merge Errors(w17, w21) -> (w19:errorcluster)
  n188 = call "Destroy User Event - Stop.vi"("error in (no error)"=w19, "User Event - Stop"=w2) -> ("error out"=w14:errorcluster)  [unwired: 9 in]
  n189 = call <vilib>:"Simple Error Handler.vi"("error in (no error)"=w14) -> ()  [unwired: 4 in, 5 out]
